vi "SensitivityV2.vi"() -> ()   [LabVIEW 2017]
uses:
  <vilib>/Analysis/1siggen.llb/Ramp Pattern by Samples.vi
  <vilib>/gmath/NI_Gmath.lvlib
  <vilib>/Analysis/NI_AALBase.lvlib
panel:
  in  "Max Output":dbl(slide) scale=0.0..10.0
  in  "Min Output":dbl(slide) scale=0.0..10.0
  out "Points":dbl[][](array[numeric])
  out "XY Graph":cluster{dbl[], dbl[]}[](graph)
  in  "Array":dbl[][](array[slide]) scale=-1.0..10.0
  in  "# of Points":i8 min=0 max=10
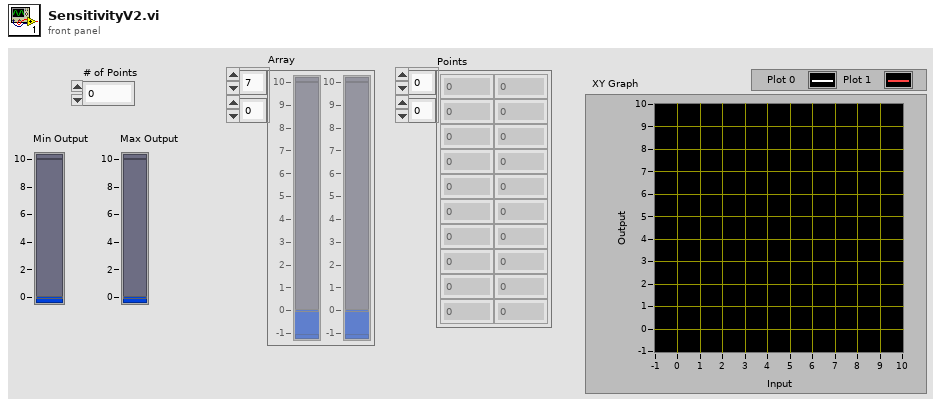
[diagram p1: front panel]
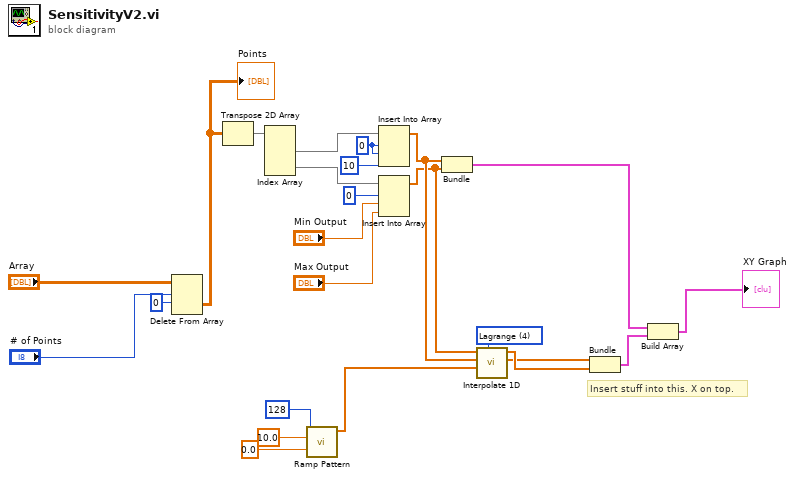
[diagram p0: block diagram]
diagram:
  w7 = 0 ("index")
  w17 = 4 items=["nearest", "linear", "spline", "cubic Hermite", "Lagrange"] ("method")
  # "Insert stuff into this. X on top."
  n1 = Delete From Array(array="Array", length="# of Points", index (row)=0) -> (deleted portion=w21:dbl[][])  [unwired: 1 in, 1 out]
  "Points" <- w21
  n2 = Transpose 2D Array(2D array=w21) -> (transposed array=w23:dbl[][])
  n3 = Index Array(array=w23) -> (element #1=w8:dbl[], element #2=w10:dbl[])  [unwired: 4 in]
  n4 = call-poly <vilib>:"Ramp Pattern.vi"("start"=0.0, "end"=10.0, "samples"=128) -> ("Ramp Pattern"=w13:dbl[])  [unwired: 7 in, 1 out]
  n5 = Insert Into Array(array=w8, index=w7, new element #1=w7, new element #2=10 ("index")) -> (w6:dbl[])
  n6 = Insert Into Array(array=w10, index=0, new element #1="Min Output", new element #2="Max Output") -> (w5:dbl[])
  n7 = Bundle(w6, w5) -> (w4:cluster{dbl[], dbl[]})  [unwired: 1 in]
  n8 = call <vilib>:"Interpolate 1D.vi"("method"=w17, "xi"=w13, "X"=w6, "Y"=w5) -> ("xi used"=w11:dbl[], "yi"=w12:dbl[])  [unwired: 5 in, 1 out]
  n9 = Bundle("xi used"=w11, "yi"=w12) -> (w18:cluster{"xi used":dbl[], "yi":dbl[]})  [unwired: 1 in]
  n10 = Build Array(w4, w18) -> (→"XY Graph":cluster{"xi used":dbl[], "yi":dbl[]}[])
